vi "TSM Site Data Calibration ID Label.vi"() -> (4 "Calibration Data Id":string)   [LabVIEW 2020]
doc: "Stores the ID Label tag for Calibration Data for TSM Site Data Variables"
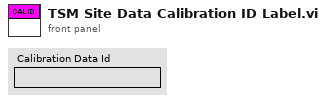
[diagram p1: front panel]
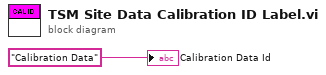
[diagram p0: block diagram]
diagram:
  "Calibration Data Id" <- "Calibration Data" ("Data Id")
